vi "Teleop Call.vi"(9 "Button Values":bool[](array[boolean])) -> ()   [LabVIEW 2017]
uses:
  Implementation/Elevator Published Globals.vi
panel:
  out "Elevator Encoder Distance":dbl
  out "Waveform Chart":dbl(graph)
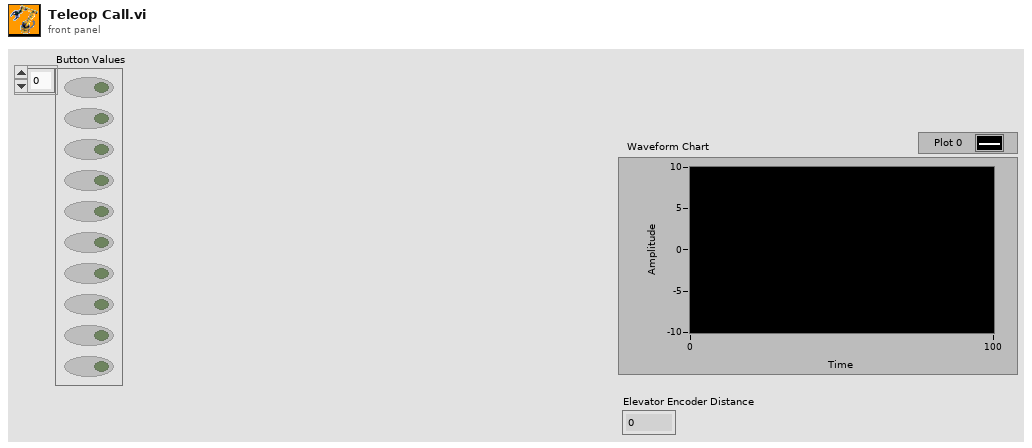
[diagram p1: front panel]
types:
  T1 = typedef "Command Status Info.ctl" = cluster{"Name":string, "Status":T2, "notifier out":T3}
  T2 = typedef "Completion Status.ctl" = enum16{"Successful", "Aborted", "Incomplete"}
  T3 = typedef "Completion Notifier.ctl" = refnum<notifier>
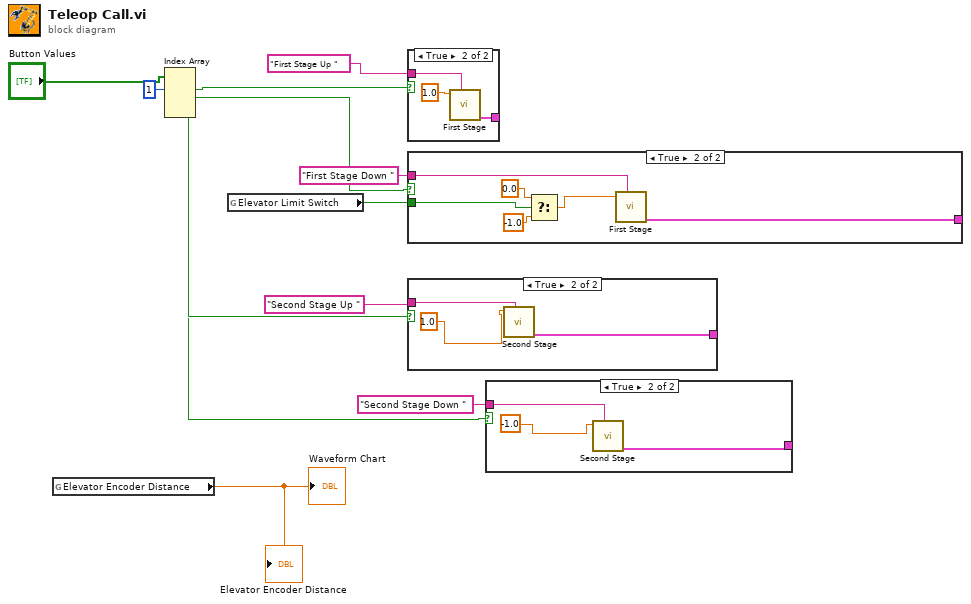
[diagram p0: block diagram]
diagram:
  n1 = global read "Elevator Published Globals.vi" "Elevator Encoder Distance"() -> (→"Waveform Chart" →"Elevator Encoder Distance":dbl)
  n2 = Index Array(array="Button Values", index #1=1 ("index")) -> (element #1=w8:bool, element #2=w7:bool, element #3=w4:bool, element #4=w3:bool)  [unwired: 3 in]
  n3 = global read "Elevator Published Globals.vi" "Elevator Limit Switch"() -> (w2:bool)
  n4 = case shown="True" w8 {
    tunnel: "First Stage Up " ("Description") -> [_ w15]
    tunnel: [_ w14] -> _
    frame False {
    }
    frame True {
      n5 = call "First Stage.vi"("Description"=w15, "Setpoint"=1.0) -> ("Command Info Out"=w14:T1)  [unwired: 9 in]
    }
  }
  n6 = case shown="True" w7 {
    tunnel: "First Stage Down " ("Description") -> [_ w21]
    tunnel: [_ w20] -> _
    tunnel: w2 -> [_ w16]
    frame False {
    }
    frame True {
      n7 = Select(t=0.0, s=w16, f=-1.0) -> (s? t:f=w18:dbl)
      n8 = call "First Stage.vi"("Description"=w21, "Setpoint"=w18) -> ("Command Info Out"=w20:T1)  [unwired: 9 in]
    }
  }
  n9 = case shown="True" w4 {
    tunnel: "Second Stage Up " ("Description") -> [_ w23]
    tunnel: [_ w22] -> _
    frame False {
    }
    frame True {
      n10 = call "Second Stage.vi"("Description"=w23, "Setpoint"=1.0) -> ("Command Info Out"=w22:T1)  [unwired: 9 in]
    }
  }
  n11 = case shown="True" w3 {
    tunnel: "Second Stage Down " ("Description") -> [_ w26]
    tunnel: [_ w25] -> _
    frame False {
    }
    frame True {
      n12 = call "Second Stage.vi"("Description"=w26, "Setpoint"=-1.0) -> ("Command Info Out"=w25:T1)  [unwired: 9 in]
    }
  }
